vi "Generate Calibration With C.vi"(0 "starting x 1":i32=100, 1 "starting y 1":i32=100, 8 "Image":T1=refnum, 14 "image In":dbl[][](array[numeric]), 15 "cross size":i32=120) -> (20 "X pos 1":dbl=111.92745564845475 format="%.2f", 21 "Y pos 1":dbl=99.9016125420082 format="%.2f", 22 "radial intensity profile 1":dbl[](array[numeric])=[155.0753564644901, 156.98257346462793, 152.10351238828963, 146.76816200641977, 136.66036950663263, 123.16471340741325, 108.27790859267813, 93.06299523045517, 77.71828799157937, 65.24345907321302, 58.81132331370246, 60.30197444351481, 70.29032042395185, 88.15116692525751, 110.56891552761617, 132.26379762825093, 147.27698227387972, 149.4935338038122, 139.16088243694125, 119.6010550063301, 99.42360774197728, 86.96391001904082, 87.54533139696333, 99.18875302385501, 114.21451481844045, 123.70107372284393, 121.53770008153512, 111.58851797544452, 101.92850705931612, 99.51165003387662, 104.79810185535041, 111.72362354943724, 113.45378152340724, 109.65600408654187, 105.10368608159517, 105.19618548353947, 109.08223587138455, 111.35917788077546, 108.96598589396633, 105.28038460072541, 105.30903108715984, 109.5643216620491, 111.95836818933167, 109.27409094506409, 104.60259060338578, 104.94946364324792, 109.79842147438394, 112.45167377247036, 108.7904792903409, 104.30773661799385, 105.49733382306134, 110.69947487726138, 112.0991469106709, 107.6462400254403, 104.28263116443613, 107.1763625707427, 111.56858068809368, 110.48834501875429, 105.73558375352992, 105.05157460683962] format="%.2f")   [LabVIEW 2014]
uses:
  <vilib>/vision/Image Controls.llb/IMAQ Image.ctl
  x64/Release/CPU Tracking.dll
panel:
  out "Waveform Graph 2":dbl[](graph)
  out "radial intensity profile 2":dbl[](array[numeric])=[155.0753564644901, 156.98257346462793, 152.10351238828963, 146.76816200641977, 136.66036950663263, 123.16471340741325, 108.27790859267813, 93.06299523045517, 77.71828799157937, 65.24345907321302, 58.81132331370246, 60.30197444351481, 70.29032042395185, 88.15116692525751, 110.56891552761617, 132.26379762825093, 147.27698227387972, 149.4935338038122, 139.16088243694125, 119.6010550063301, 99.42360774197728, 86.96391001904082, 87.54533139696333, 99.18875302385501, 114.21451481844045, 123.70107372284393, 121.53770008153512, 111.58851797544452, 101.92850705931612, 99.51165003387662, 104.79810185535041, 111.72362354943724, 113.45378152340724, 109.65600408654187, 105.10368608159517, 105.19618548353947, 109.08223587138455, 111.35917788077546, 108.96598589396633, 105.28038460072541, 105.30903108715984, 109.5643216620491, 111.95836818933167, 109.27409094506409, 104.60259060338578, 104.94946364324792, 109.79842147438394, 112.45167377247036, 108.7904792903409, 104.30773661799385, 105.49733382306134, 110.69947487726138, 112.0991469106709, 107.6462400254403, 104.28263116443613, 107.1763625707427, 111.56858068809368, 110.48834501875429, 105.73558375352992, 105.05157460683962] format="%.2f"
  out "Waveform Graph":dbl[](graph)
  out "Image 2":T1(plugin-control)
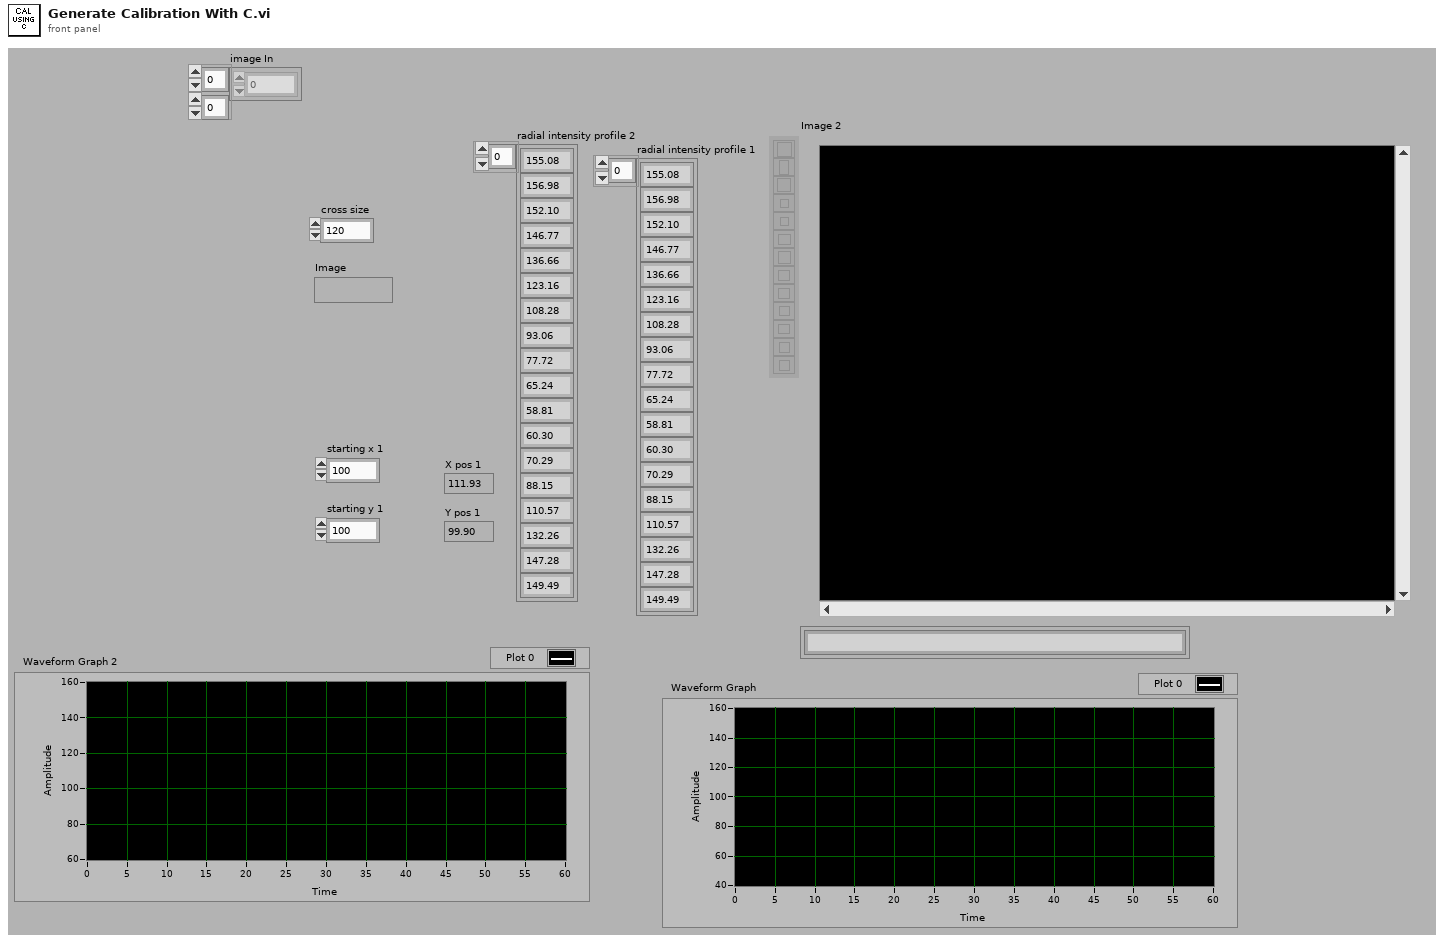
[diagram p1: front panel]
types:
  T1 = typedef "IMAQ Image.ctl" = refnum<image>
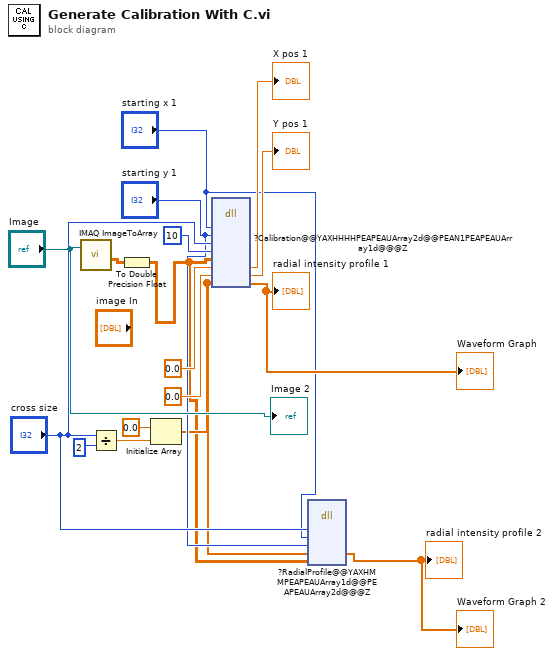
[diagram p0: block diagram]
diagram:
  n1 = call "IMAQ ImageToArray"("Image"="Image") -> ("Image Pixels (Float)"=w2:sgl[][])  [unwired: 3 in, 4 out]
  n2 = Divide(x="cross size", y=2) -> (x/y=w16:dbl)
  n3 = To Double Precision Float(number=w2) -> (double precision float=w1:dbl[][])
  n4 = Initialize Array(0.0 ("element"), w16) -> (w4:dbl[])
  n5 = dll-call lib="D:/LV-SVN/Projects/Bob/GPU Tracking Demo/CPU Tracking & Calibration/x64/Release/CPU Tracking.dll" fn="?Calibration@@YAXHHHHPEAPEAUArray2d@@PEAN1PEAPEAUArray1d@@@Z"("x"="starting x 1", "y"="starting y 1", "cross"="cross size", "crossthickness"=10 ("cross arm width"), "image"=w1, "xout"=0.0, "yout"=0.0, "RadProfileOut"=w4) -> ("xout"=→"X pos 1":dbl, "yout"=→"Y pos 1":dbl, "RadProfileOut"=→"radial intensity profile 1" →"Waveform Graph":dbl[])  [unwired: 9 in, 2 out]
  n6 = dll-call lib="D:/LV-SVN/Projects/Bob/GPU Tracking Demo/CPU Tracking & Calibration/x64/Release/CPU Tracking.dll" fn="?RadialProfile@@YAXHMMPEAPEAUArray1d@@PEAPEAUArray2d@@@Z"("cross"="cross size", "x"="starting x 1", "y"="starting y 1", "RadProfileOut"=w4, "image"=w1) -> ("RadProfileOut"=→"radial intensity profile 2" →"Waveform Graph 2":dbl[])  [unwired: 8 in, 2 out]
  "Image 2" <- "Image"
